vi "Error Logger.vi"(8 "error in (no error)":errorcluster, 10 "Logging Directory":path) -> (0 "error out":errorcluster)   [LabVIEW 2009]
uses:
  <vilib>/Utility/error.llb/DialogType.ctl
panel:
  in  "Error Log Filename":string="Operations Manager Program Errors.txt"
  out "Message":string
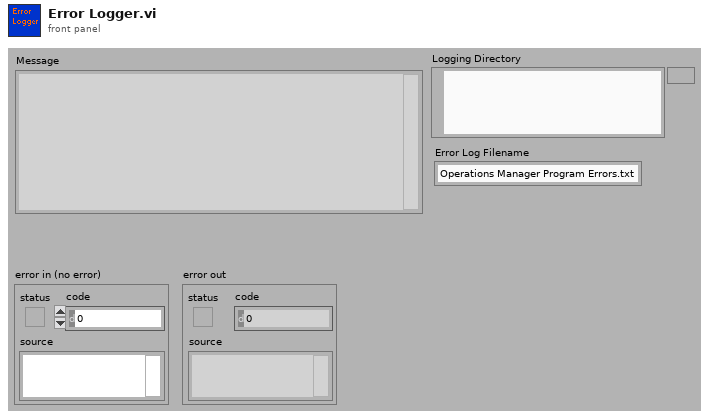
[diagram p1: front panel]
types:
  T1 = enum16{"open", "replace", "create", "open or create", "replace or create", "replace or create with confirmation"}
  T2 = typedef "DialogType.ctl" = u16
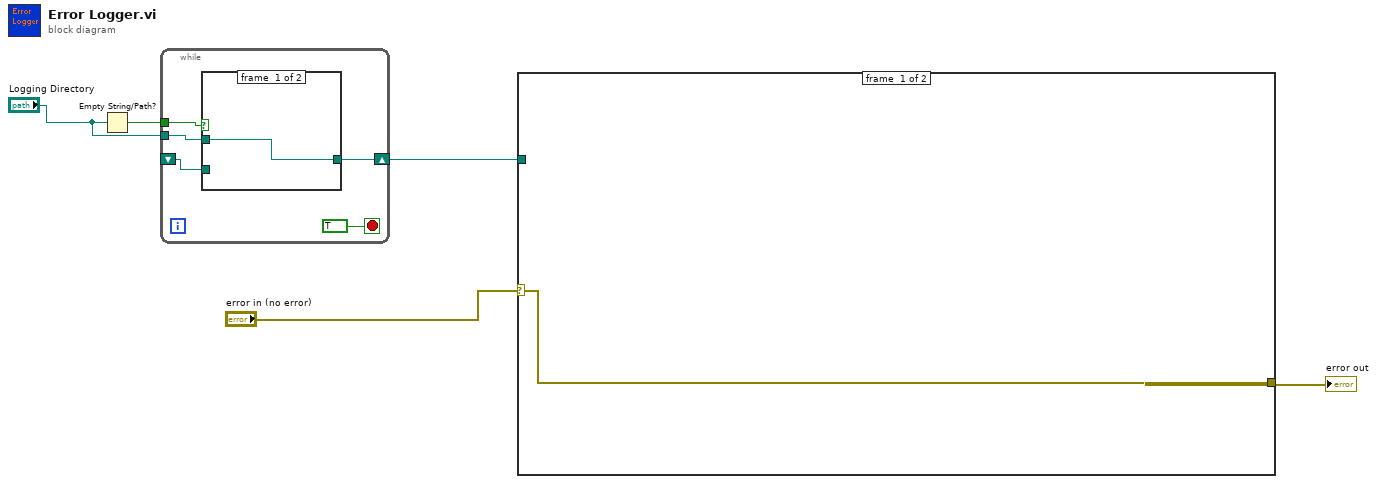
[diagram p0: block diagram]
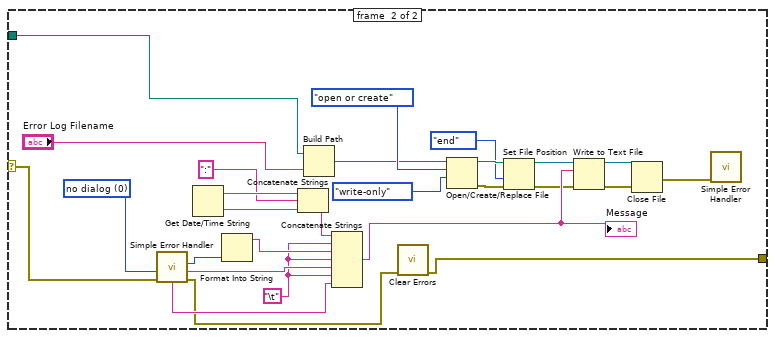
[diagram p3: hidden frame]
diagram:
  n1 = Empty String/Path?(string/path="Logging Directory") -> (empty?=w2:bool)
  n2 = while {
    tunnel: w2 -> [w8]
    tunnel: "Logging Directory" -> [w7]
    shift-right: [w9] -> w3
    shift-left: _ -> [w6]
    stop <- TRUE stop-if-true
    n3 = case shown="True" w8 {
      tunnel: [w11 w12] -> w9
      tunnel: w7 -> [w11 _]
      tunnel: w6 -> [_ w12]
      frame #0 {
      }
      frame #1 {
      }
    }
  }
  n4 = case shown="Error" "error in (no error)" {
    selector: "error in (no error)" -> [w13 w24]
    tunnel: [w13 w31] -> w5
    tunnel: w3 -> [_ w14]
    frame #0 {
    }
    frame #1 {
      w15 = T2 0 items=["no dialog", "OK message", "continue or stop message", "OK message + warnings", "continue/stop + warnings"] ("type of dialog (OK msg:1)")
      w25 = "\t"
      n5 = call <vilib>:"Simple Error Handler.vi"("type of dialog (OK msg:1)"=w15, "error in (no error)"=w24) -> ("code out"=w36:i32, "source out"=w34:string, "error out"=w32:errorcluster, "message"=w33:string)  [unwired: 4 out]
      n6 = Get Date/Time String() -> (date string=w29:string, time string=w28:string)  [unwired: 3 out]
      n7 = Format Into String(w36) -> (resulting string=w35:string)  [unwired: 3 in, 1 out]
      n8 = Concatenate Strings(w29, ":" ("string"), w28) -> (w26:string)
      n9 = Build Path(base path=w14, name or relative path="Error Log Filename") -> (appended path=w20:path)
      n10 = Concatenate Strings(w26, w25, w35, w25, w34, w25, w33) -> (w30:string)
      "Message" <- w30
      n11 = call <vilib>:"Clear Errors.vi"("error in (no error)"=w32) -> ("error out"=w31:errorcluster)  [unwired: 6 out]
      n12 = Open/Create/Replace File(file path (use dialog)=w20, operation (0:open)=T1."open or create", access (0:read/write)=enum16{"read/write", "read-only", "write-only"}."write-only") -> (refnum out=w38:refnum<file>, error out=w18:errorcluster)  [unwired: 1 in, 3 out]
      n13 = Set File Position(refnum=w38, from (0:start)=enum16{"start", "end", "current"}."end", error in=w18) -> (refnum out=w19:refnum<file>, error out=w16:errorcluster)  [unwired: 1 out]
      n14 = Write to Text File(file (use dialog)=w19, text=w30, error in=w16) -> (refnum out=w37:refnum<file>, error out=w23:errorcluster)  [unwired: 2 out]
      n15 = Close File(refnum=w37, error in=w23) -> (error out=w22:errorcluster)  [unwired: 1 out]
      n16 = call <vilib>:"Simple Error Handler.vi"("error in (no error)"=w22) -> ()  [unwired: 1 in, 8 out]
    }
  }
  "error out" <- w5
